vi "fuzzyex Simulate Car position.vi"(4 "方向":bool, 6 "转向角(Phi)":dbl format="%.2f", 7 "当前车辆方位(Beta)":dbl format="%.2f", 8 "当前位置Y":dbl format="%.2f", 9 "当前位置X":dbl format="%.2f") -> (1 "新车辆方位(Beta)":dbl format="%.2f", 2 "新位置Y":dbl format="%.2f", 3 "新位置X":dbl format="%.2f")   [LabVIEW 2018]
doc: "本VI在车辆行驶控制模型中用来计算车辆新位置（车辆中心的X(VC)和Y(VC)坐标）、给定转向角(Phi)的车辆车辆方位(Beta)、移动方向（方向：＝前进｜后退）。"
panel:
  # "移动方向（关＝后退）"
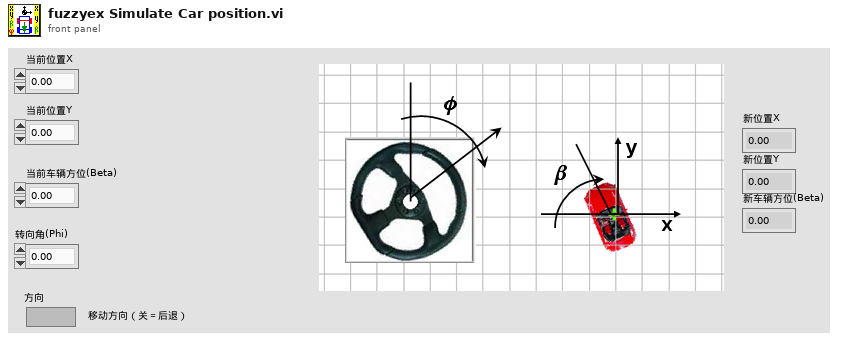
[diagram p1: front panel]
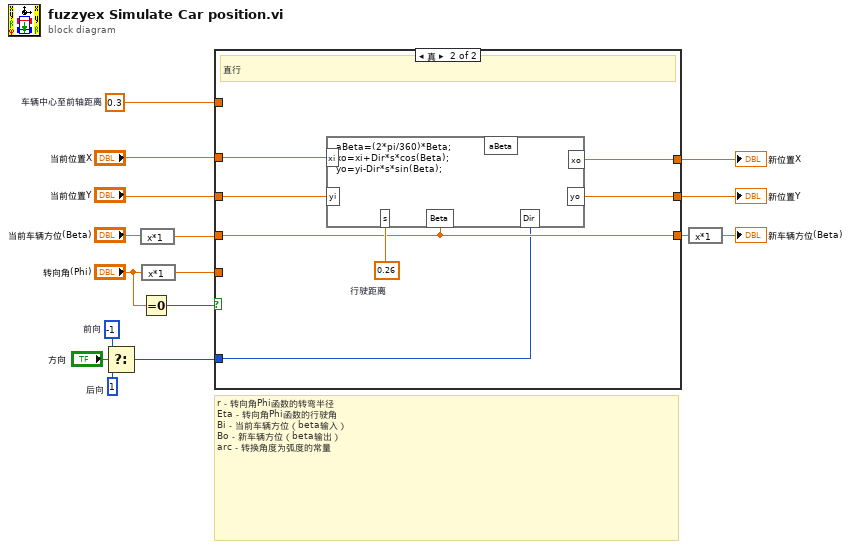
[diagram p0: block diagram]
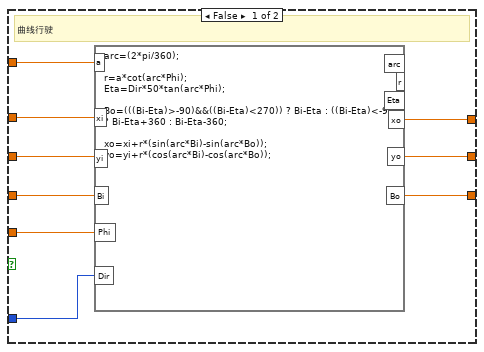
[diagram p2: hidden frame]
diagram:
  w1 = 0.3  # 车辆中心至前轴距离
  w9 = -1  # 前向
  w8 = 1  # 后向
  # "r－转向角Phi函数的转弯半径\nEta－转向角Phi函数的行驶角\nBi－当前车辆方位（beta输入）\nBo－新车辆方位（beta输出）\narc－转换角度为弧度的常量"
  n1 = Select(t=w9, s="方向", f=w8) -> (s? t:f=w7:i32)
  n2 = expression code="x*1"("当前车辆方位(Beta)") -> (w5:dbl)
  n3 = Equal To 0?(x="转向角(Phi)") -> (x = 0?=w16:bool)
  n4 = expression code="x*1"("转向角(Phi)") -> (w6:dbl)
  n5 = case shown="真" w16 {
    tunnel: w5 -> [w23 w31]
    tunnel: [w21 w31] -> w3
    tunnel: "当前位置X" -> [w25 w30]
    tunnel: "当前位置Y" -> [w24 w29]
    tunnel: [w20 w28] -> w13
    tunnel: [w22 w27] -> w12
    tunnel: w6 -> [w19 _]
    tunnel: w7 -> [w18 w26]
    tunnel: w1 -> [w17 _]
    frame False {
      # "曲线行驶"
      n6 = formula code="arc=(2*pi/360);\n\nr=a*cot(arc*Phi);\nEta=Dir*50*tan(arc*Phi);\n\nBo=(((Bi-Eta)>-90)&&((Bi-Eta)<270)) ? Bi-Eta : ((Bi-Eta)<-90) ? Bi-Eta+360 : Bi-Eta-360;\n\nxo=xi+r*(sin(arc*Bi)-sin(arc*Bo));\nyo=yi+r*(cos(arc*Bi)-cos(arc*Bo));"("xi"=w25, "yi"=w24, "Bi"=w23, "Phi"=w19, "a"=w17, "Dir"=w18) -> ("yo"=w22:dbl, "Bo"=w21:dbl, "xo"=w20:dbl)  [unwired: 3 out]
    }
    frame True {
      w32 = 0.26  # 行驶距离
      # "直行"
      n7 = formula code="aBeta=(2*pi/360)*Beta;\nxo=xi+Dir*s*cos(Beta);\nyo=yi-Dir*s*sin(Beta);"("xi"=w30, "yi"=w29, "s"=w32, "Beta"=w31, "Dir"=w26) -> ("xo"=w28:dbl, "yo"=w27:dbl)  [unwired: 1 out]
    }
  }
  "新位置X" <- w13
  "新位置Y" <- w12
  n8 = expression code="x*1"(w3) -> (→"新车辆方位(Beta)":dbl)
